vi "SimpleImport.vi"() -> ()   [LabVIEW 2019]
uses:
  <userlib>/MicroPython/VIs/uPythonX/uPythonX.xctl
panel:
  in  "fred":T1(xcontrol)={"VISA Refnum in"="ASRL44::INSTR", "Python Code"="def hello():\n     print ('hello')"}
  in  "uPythonX":T1(xcontrol)={"VISA Refnum in"="ASRL44::INSTR", "Python Code"="import fred\nfred.hello()"}
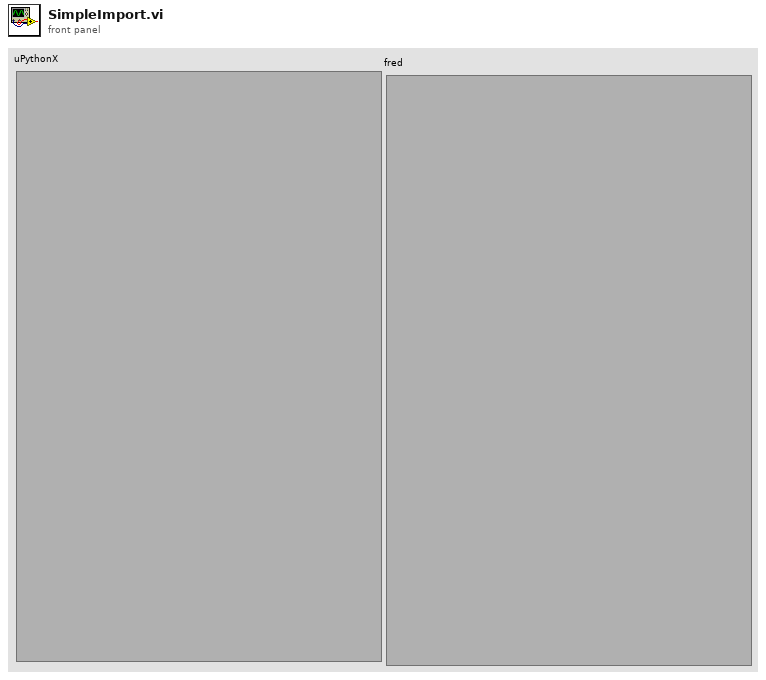
[diagram p1: front panel]
types:
  T1 = cluster{"VISA Refnum in":refnum<visa-resource-name>, "Python Code":string}
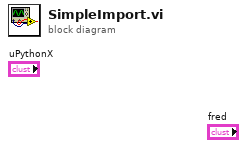
[diagram p0: block diagram]
diagram:
